vi "Read Behavior.vi"(11 "Filter in":refnum<class "Filter.lvclass">) -> (2 "match behavior":T1, 3 "Filter out":refnum<class "Filter.lvclass">)   [LabVIEW 2018, in "GLog.lvlib" / "Filter.lvclass"]
uses:
  Filter.lvclass
  Match Behavior.ctl
  Filter.lvclass/Filter.ctl
  GLog.lvlib
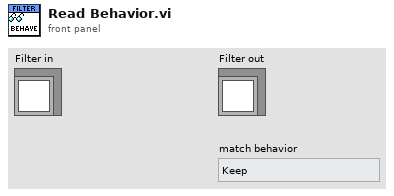
[diagram p1: front panel]
types:
  T1 = typedef "GLog.lvlib/Match Behavior.ctl" = enum16{"Keep", "Discard"}
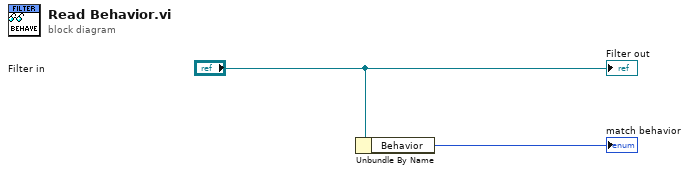
[diagram p0: block diagram]
diagram:
  n1 = Unbundle By Name("Filter in") -> ("Behavior"=→"match behavior":T1)
  "Filter out" <- "Filter in"
